vi "test-Mecanum-Kinematics-Test1.vi"() -> (3 "All tests passed":bool)   [LabVIEW 2019]
uses:
  <vilib>/Rock Robotics/WPI/ThirdParty/JAS_Junk/TrajLib/Trajectory_Library.lvlib
panel:
  out "Test 13":bool
  out "Test 12":bool
  out "Test 11":bool
  out "Test 10":bool
  out "Test 9":bool
  out "Test 8":bool
  out "Test 7":bool
  out "Test 6":bool
  out "Test 5":bool
  out "Test 4":bool
  out "Test 3":bool
  out "Test 2":bool
  out "Test 1":bool
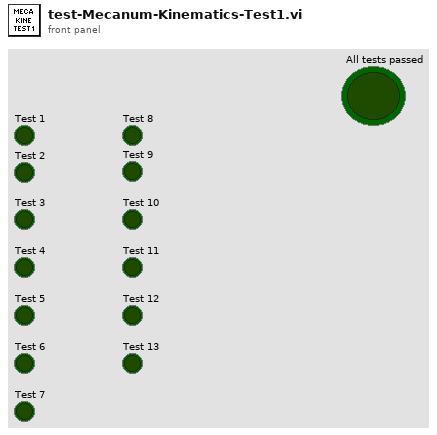
[diagram p1: front panel]
types:
  T1 = typedef "Trajectory_Library.lvlib/TRANSLATION2D.ctl" = cluster{"X":dbl, "Y":dbl}
  T2 = typedef "Trajectory_Library.lvlib/MECA_WHEEL_SPEEDS.ctl" = cluster{"FrontLeftSpeed":dbl, "FrontRightSpeed":dbl, "RearLeftSpeed":dbl, "RearRightSpeed":dbl}
  T3 = typedef "Trajectory_Library.lvlib/CHASSIS_SPEEDS.ctl" = cluster{"vX":dbl, "vY":dbl, "vOmega":dbl}
  T4 = typedef "Trajectory_Library.lvlib/MECA_DRIVE_KINEMATICS.ctl" = cluster{"FrontLeft":T1, "FrontRight":T1, "RearLeft":T1, "RearRight":T1, "InverseKinematics":T5, "ForwardKinematics":T5, "PrevCoR":T1}
  T5 = typedef "NI_Matrix.lvlib/RealMatrix.ctl" = dbl[][]
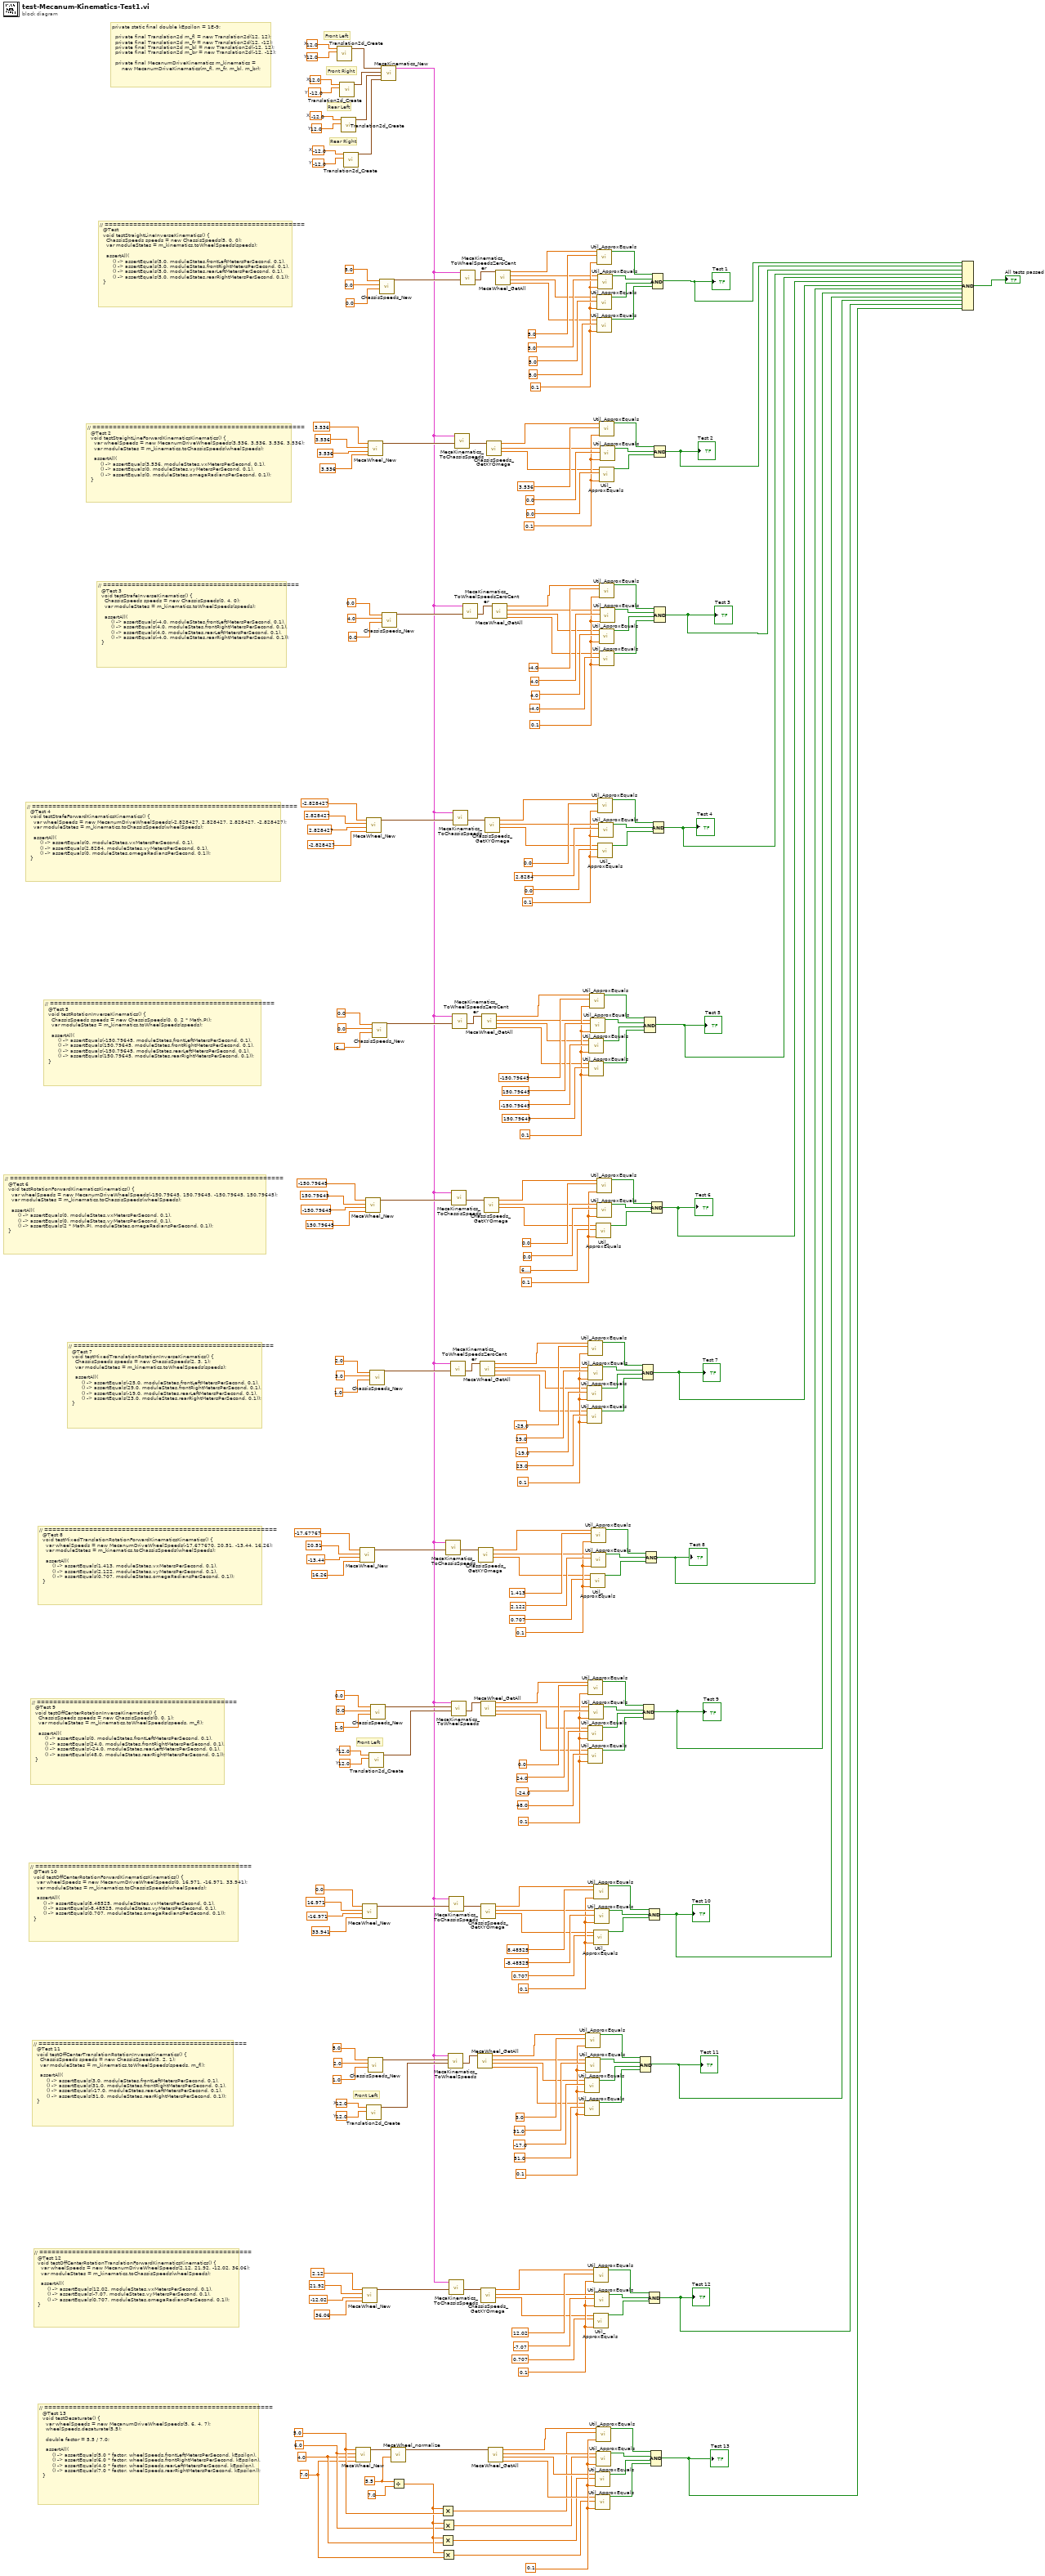
[diagram p0: block diagram]
diagram:
  w11 = 0.1 ("Tolerance")
  w22 = 5.5 ("MaxAttainableSpeed")
  w20 = 5.0 ("FrontLeftSpeed")
  w18 = 6.0 ("FrontRightSpeed")
  w17 = 4.0 ("RearLeftSpeed")
  w16 = 7.0 ("RearRightSpeed")
  w30 = 0.1 ("Tolerance")
  w46 = 12.0  # X
  w44 = 12.0  # Y
  w53 = 0.1 ("Tolerance")
  w67 = 0.1 ("Tolerance")
  w84 = 12.0  # X
  w82 = 12.0  # Y
  w91 = 0.1 ("Tolerance")
  w111 = 0.1 ("Tolerance")
  w131 = 0.1 ("Tolerance")
  w145 = 0.1 ("Tolerance")
  w165 = 0.1 ("Tolerance")
  w178 = 0.1 ("Tolerance")
  w204 = 0.1 ("Tolerance")
  w205 = 0.1 ("Tolerance")
  w206 = 0.1 ("Tolerance")
  w251 = -12.0  # X
  w250 = -12.0  # Y
  w249 = -12.0  # X
  w248 = 12.0  # Y
  w247 = 12.0  # X
  w246 = -12.0  # Y
  w245 = 12.0  # X
  w244 = 12.0  # Y
  # "// ========================================================\n  @Test 13\n  void testDesaturate() {\n    var wheelSpeeds = new MecanumDriveWheelSpeeds(5, 6, 4, 7);\n    wheelSpeeds.desaturate(5.5);\n\n    double factor = 5.5 / 7.0;\n\n    assertAll(\n        () -> assertEquals(5.0 * factor, wheelSpeeds.frontLeftMetersPerSecond, kEpsilon),\n        () -> assertEquals(6.0 * factor, wheelSpeeds.frontRightMetersPerSecond, kEpsilon),\n        () -> assertEquals(4.0 * factor, wheelSpeeds.rearLeftMetersPerSecond, kEpsilon),\n        () -> assertEquals(7.0 * factor, wheelSpeeds.rearRightMetersPerSecond, kEpsilon));\n  }"
  # "// ====================================================\n  @Test 12\n  void testOffCenterRotationTranslationForwardKinematicsKinematics() {\n    var wheelSpeeds = new MecanumDriveWheelSpeeds(2.12, 21.92, -12.02, 36.06);\n    var moduleStates = m_kinematics.toChassisSpeeds(wheelSpeeds);\n\n    assertAll(\n        () -> assertEquals(12.02, moduleStates.vxMetersPerSecond, 0.1),\n        () -> assertEquals(-7.07, moduleStates.vyMetersPerSecond, 0.1),\n        () -> assertEquals(0.707, moduleStates.omegaRadiansPerSecond, 0.1));\n  }"
  # "// ===================================================\n  @Test 11\n  void testOffCenterTranslationRotationInverseKinematics() {\n    ChassisSpeeds speeds = new ChassisSpeeds(5, 2, 1);\n    var moduleStates = m_kinematics.toWheelSpeeds(speeds, m_fl);\n\n    assertAll(\n        () -> assertEquals(3.0, moduleStates.frontLeftMetersPerSecond, 0.1),\n        () -> assertEquals(31.0, moduleStates.frontRightMetersPerSecond, 0.1),\n        () -> assertEquals(-17.0, moduleStates.rearLeftMetersPerSecond, 0.1),\n        () -> assertEquals(51.0, moduleStates.rearRightMetersPerSecond, 0.1));\n  }"
  # "Front Left"
  # "// =====================================================\n  @Test 10\n  void testOffCenterRotationForwardKinematicsKinematics() {\n    var wheelSpeeds = new MecanumDriveWheelSpeeds(0, 16.971, -16.971, 33.941);\n    var moduleStates = m_kinematics.toChassisSpeeds(wheelSpeeds);\n\n    assertAll(\n        () -> assertEquals(8.48525, moduleStates.vxMetersPerSecond, 0.1),\n        () -> assertEquals(-8.48525, moduleStates.vyMetersPerSecond, 0.1),\n        () -> assertEquals(0.707, moduleStates.omegaRadiansPerSecond, 0.1));\n  }"
  # "Front Left"
  # "// =================================================\n  @Test 9\n  void testOffCenterRotationInverseKinematics() {\n    ChassisSpeeds speeds = new ChassisSpeeds(0, 0, 1);\n    var moduleStates = m_kinematics.toWheelSpeeds(speeds, m_fl);\n\n    assertAll(\n        () -> assertEquals(0, moduleStates.frontLeftMetersPerSecond, 0.1),\n        () -> assertEquals(24.0, moduleStates.frontRightMetersPerSecond, 0.1),\n        () -> assertEquals(-24.0, moduleStates.rearLeftMetersPerSecond, 0.1),\n        () -> assertEquals(48.0, moduleStates.rearRightMetersPerSecond, 0.1));\n  }"
  # "// =========================================================\n  @Test 8\n  void testMixedTranslationRotationForwardKinematicsKinematics() {\n    var wheelSpeeds = new MecanumDriveWheelSpeeds(-17.677670, 20.51, -13.44, 16.26);\n    var moduleStates = m_kinematics.toChassisSpeeds(wheelSpeeds);\n\n    assertAll(\n        () -> assertEquals(1.413, moduleStates.vxMetersPerSecond, 0.1),\n        () -> assertEquals(2.122, moduleStates.vyMetersPerSecond, 0.1),\n        () -> assertEquals(0.707, moduleStates.omegaRadiansPerSecond, 0.1));\n  }"
  # "// =================================================\n  @Test 7\n  void testMixedTranslationRotationInverseKinematics() {\n    ChassisSpeeds speeds = new ChassisSpeeds(2, 3, 1);\n    var moduleStates = m_kinematics.toWheelSpeeds(speeds);\n\n    assertAll(\n        () -> assertEquals(-25.0, moduleStates.frontLeftMetersPerSecond, 0.1),\n        () -> assertEquals(29.0, moduleStates.frontRightMetersPerSecond, 0.1),\n        () -> assertEquals(-19.0, moduleStates.rearLeftMetersPerSecond, 0.1),\n        () -> assertEquals(23.0, moduleStates.rearRightMetersPerSecond, 0.1));\n  }"
  # "// ===================================================================\n  @Test 6\n  void testRotationForwardKinematicsKinematics() {\n    var wheelSpeeds = new MecanumDriveWheelSpeeds(-150.79645, 150.79645, -150.79645, 150.79645);\n    var moduleStates = m_kinematics.toChassisSpeeds(wheelSpeeds);\n\n    assertAll(\n        () -> assertEquals(0, moduleStates.vxMetersPerSecond, 0.1),\n        () -> assertEquals(0, moduleStates.vyMetersPerSecond, 0.1),\n        () -> assertEquals(2 * Math.PI, moduleStates.omegaRadiansPerSecond, 0.1));\n  }"
  # "// =======================================================\n  @Test 5\n  void testRotationInverseKinematics() {\n    ChassisSpeeds speeds = new ChassisSpeeds(0, 0, 2 * Math.PI);\n    var moduleStates = m_kinematics.toWheelSpeeds(speeds);\n\n    assertAll(\n        () -> assertEquals(-150.79645, moduleStates.frontLeftMetersPerSecond, 0.1),\n        () -> assertEquals(150.79645, moduleStates.frontRightMetersPerSecond, 0.1),\n        () -> assertEquals(-150.79645, moduleStates.rearLeftMetersPerSecond, 0.1),\n        () -> assertEquals(150.79645, moduleStates.rearRightMetersPerSecond, 0.1));\n  }"
  # "// =================================================================\n  @Test 4\n  void testStrafeForwardKinematicsKinematics() {\n    var wheelSpeeds = new MecanumDriveWheelSpeeds(-2.828427, 2.828427, 2.828427, -2.828427);\n    var moduleStates = m_kinematics.toChassisSpeeds(wheelSpeeds);\n\n    assertAll(\n        () -> assertEquals(0, moduleStates.vxMetersPerSecond, 0.1),\n        () -> assertEquals(2.8284, moduleStates.vyMetersPerSecond, 0.1),\n        () -> assertEquals(0, moduleStates.omegaRadiansPerSecond, 0.1));\n  }"
  # "// ================================================\n  @Test 3\n  void testStrafeInverseKinematics() {\n    ChassisSpeeds speeds = new ChassisSpeeds(0, 4, 0);\n    var moduleStates = m_kinematics.toWheelSpeeds(speeds);\n\n    assertAll(\n        () -> assertEquals(-4.0, moduleStates.frontLeftMetersPerSecond, 0.1),\n        () -> assertEquals(4.0, moduleStates.frontRightMetersPerSecond, 0.1),\n        () -> assertEquals(4.0, moduleStates.rearLeftMetersPerSecond, 0.1),\n        () -> assertEquals(-4.0, moduleStates.rearRightMetersPerSecond, 0.1));\n  }"
  # "// ====================================================\n  @Test 2\n  void testStraightLineForwardKinematicsKinematics() {\n    var wheelSpeeds = new MecanumDriveWheelSpeeds(3.536, 3.536, 3.536, 3.536);\n    var moduleStates = m_kinematics.toChassisSpeeds(wheelSpeeds);\n\n    assertAll(\n        () -> assertEquals(3.536, moduleStates.vxMetersPerSecond, 0.1),\n        () -> assertEquals(0, moduleStates.vyMetersPerSecond, 0.1),\n        () -> assertEquals(0, moduleStates.omegaRadiansPerSecond, 0.1));\n  }"
  # "Rear Right"
  # "Rear Left"
  # "Front Right"
  # "Front Left"
  # "private static final double kEpsilon = 1E-9;\n\n  private final Translation2d m_fl = new Translation2d(12, 12);\n  private final Translation2d m_fr = new Translation2d(12, -12);\n  private final Translation2d m_bl = new Translation2d(-12, 12);\n  private final Translation2d m_br = new Translation2d(-12, -12);\n\n  private final MecanumDriveKinematics m_kinematics =\n      new MecanumDriveKinematics(m_fl, m_fr, m_bl, m_br);"
  # "// =================================================\n  @Test\n  void testStraightLineInverseKinematics() {\n    ChassisSpeeds speeds = new ChassisSpeeds(5, 0, 0);\n    var moduleStates = m_kinematics.toWheelSpeeds(speeds);\n\n    assertAll(\n        () -> assertEquals(5.0, moduleStates.frontLeftMetersPerSecond, 0.1),\n        () -> assertEquals(5.0, moduleStates.frontRightMetersPerSecond, 0.1),\n        () -> assertEquals(5.0, moduleStates.rearLeftMetersPerSecond, 0.1),\n        () -> assertEquals(5.0, moduleStates.rearRightMetersPerSecond, 0.1));\n  }"
  n1 = call <vilib>:"Translation2d_Create.vi"("Y"=w244, "X"=w245) -> ("TRANSLATION"=w252:T1)  [unwired: 9 in]
  n2 = call <vilib>:"Translation2d_Create.vi"("Y"=w246, "X"=w247) -> ("TRANSLATION"=w253:T1)  [unwired: 9 in]
  n3 = call <vilib>:"Translation2d_Create.vi"("Y"=w248, "X"=w249) -> ("TRANSLATION"=w254:T1)  [unwired: 9 in]
  n4 = call <vilib>:"Translation2d_Create.vi"("Y"=w250, "X"=w251) -> ("TRANSLATION"=w255:T1)  [unwired: 9 in]
  n5 = call <vilib>:"MecaWheel_New.vi"("RearRightSpeed"=w16, "RearLeftSpeed"=w17, "FrontRightSpeed"=w18, "FrontLeftSpeed"=w20) -> ("MECA_WHEEL_SPEEDS"=w23:T2)  [unwired: 7 in]
  n6 = call <vilib>:"MecaWheel_New.vi"("RearRightSpeed"=16.26, "RearLeftSpeed"=-13.44, "FrontRightSpeed"=20.51, "FrontLeftSpeed"=-17.67767) -> ("MECA_WHEEL_SPEEDS"=w115:T2)  [unwired: 7 in]
  n7 = call <vilib>:"MecaWheel_New.vi"("RearRightSpeed"=33.941, "RearLeftSpeed"=-16.971, "FrontRightSpeed"=16.971, "FrontLeftSpeed"=0.0) -> ("MECA_WHEEL_SPEEDS"=w71:T2)  [unwired: 7 in]
  n8 = call <vilib>:"MecaWheel_New.vi"("RearRightSpeed"=36.06, "RearLeftSpeed"=-12.02, "FrontRightSpeed"=21.92, "FrontLeftSpeed"=2.12) -> ("MECA_WHEEL_SPEEDS"=w34:T2)  [unwired: 7 in]
  n9 = call <vilib>:"MecaWheel_New.vi"("RearRightSpeed"=150.79645, "RearLeftSpeed"=-150.79645, "FrontRightSpeed"=150.79645, "FrontLeftSpeed"=-150.79645) -> ("MECA_WHEEL_SPEEDS"=w149:T2)  [unwired: 7 in]
  n10 = call <vilib>:"Translation2d_Create.vi"("Y"=w44, "X"=w46) -> ("TRANSLATION"=w45:T1)  [unwired: 9 in]
  n11 = call <vilib>:"MecaWheel_New.vi"("RearRightSpeed"=-2.828427, "RearLeftSpeed"=2.828427, "FrontRightSpeed"=2.828427, "FrontLeftSpeed"=-2.828427) -> ("MECA_WHEEL_SPEEDS"=w182:T2)  [unwired: 7 in]
  n12 = call <vilib>:"ChassisSpeeds_New.vi"("vAngular"=1.0 ("vX"), "vY"=2.0, "vX"=5.0) -> ("CHASSIS"=w27:T3)  [unwired: 8 in]
  n13 = call <vilib>:"MecaWheel_New.vi"("RearRightSpeed"=3.536, "RearLeftSpeed"=3.536, "FrontRightSpeed"=3.536, "FrontLeftSpeed"=3.536) -> ("MECA_WHEEL_SPEEDS"=w223:T2)  [unwired: 7 in]
  n14 = call <vilib>:"Translation2d_Create.vi"("Y"=w82, "X"=w84) -> ("TRANSLATION"=w83:T1)  [unwired: 9 in]
  n15 = call <vilib>:"ChassisSpeeds_New.vi"("vAngular"=1.0 ("vX"), "vY"=3.0, "vX"=2.0) -> ("CHASSIS"=w140:T3)  [unwired: 8 in]
  n16 = call <vilib>:"ChassisSpeeds_New.vi"("vAngular"=1.0 ("vX"), "vY"=0.0, "vX"=0.0) -> ("CHASSIS"=w100:T3)  [unwired: 8 in]
  n17 = call <vilib>:"ChassisSpeeds_New.vi"("vAngular"=6.283185307179586, "vY"=0.0, "vX"=0.0) -> ("CHASSIS"=w174:T3)  [unwired: 8 in]
  n18 = call <vilib>:"ChassisSpeeds_New.vi"("vAngular"=0.0, "vY"=0.0, "vX"=5.0) -> ("CHASSIS"=w243:T3)  [unwired: 8 in]
  n19 = call <vilib>:"MecaKinematics_New.vi"("RearRight"=w255, "RearLeft"=w254, "FrontRight"=w253, "FrontLeft"=w252) -> ("MECA_DRIVE_KINEMATICS"=w26:T4)  [unwired: 7 in]
  n20 = call <vilib>:"ChassisSpeeds_New.vi"("vAngular"=0.0, "vY"=4.0, "vX"=0.0) -> ("CHASSIS"=w215:T3)  [unwired: 8 in]
  n21 = call <vilib>:"MecaWheel_normalize.vi"("MaxAttainableSpeed"=w22, "in MECA_WHEEL_SPEEDS"=w23) -> ("out MECA_WHEEL_SPEEDS"=w6:T2)  [unwired: 9 in]
  n22 = Divide(x=w22, y=7.0) -> (x/y=w19:dbl)
  n23 = Multiply(x=w19, y=w20) -> (x*y=w5:dbl)
  n24 = Multiply(x=w19, y=w17) -> (x*y=w3:dbl)
  n25 = Multiply(x=w19, y=w18) -> (x*y=w4:dbl)
  n26 = Multiply(x=w19, y=w16) -> (x*y=w2:dbl)
  n27 = call <vilib>:"MecaKinematics_ToChassisSpeeds.vi"("MECA_WHEEL_SPEEDS"=w115, "in MECA_DRIVE_KINEMATICS"=w26) -> ("ChassisSpeeds"=w114:T3)  [unwired: 9 in]
  n28 = call <vilib>:"MecaKinematics_ToWheelSpeeds.vi"("CenterOfRotation"=w45, "ChassisSpeeds"=w27, "in MECA_DRIVE_KINEMATICS"=w26) -> ("MECA_WHEEL_SPEEDS"=w52:T2)  [unwired: 7 in, 1 out]
  n29 = call <vilib>:"MecaKinematics_ToChassisSpeeds.vi"("MECA_WHEEL_SPEEDS"=w71, "in MECA_DRIVE_KINEMATICS"=w26) -> ("ChassisSpeeds"=w70:T3)  [unwired: 9 in]
  n30 = call <vilib>:"MecaKinematics_ToChassisSpeeds.vi"("MECA_WHEEL_SPEEDS"=w34, "in MECA_DRIVE_KINEMATICS"=w26) -> ("ChassisSpeeds"=w33:T3)  [unwired: 9 in]
  n31 = call <vilib>:"MecaKinematics_ToWheelSpeedsZeroCenter.vi"("ChassisSpeeds"=w140, "in MECA_DRIVE_KINEMATICS"=w26) -> ("MECA_WHEEL_SPEEDS"=w130:T2)  [unwired: 8 in, 1 out]
  n32 = call <vilib>:"MecaKinematics_ToWheelSpeeds.vi"("CenterOfRotation"=w83, "ChassisSpeeds"=w100, "in MECA_DRIVE_KINEMATICS"=w26) -> ("MECA_WHEEL_SPEEDS"=w90:T2)  [unwired: 7 in, 1 out]
  n33 = call <vilib>:"MecaKinematics_ToChassisSpeeds.vi"("MECA_WHEEL_SPEEDS"=w149, "in MECA_DRIVE_KINEMATICS"=w26) -> ("ChassisSpeeds"=w148:T3)  [unwired: 9 in]
  n34 = call <vilib>:"MecaKinematics_ToWheelSpeedsZeroCenter.vi"("ChassisSpeeds"=w174, "in MECA_DRIVE_KINEMATICS"=w26) -> ("MECA_WHEEL_SPEEDS"=w164:T2)  [unwired: 8 in, 1 out]
  n35 = call <vilib>:"MecaKinematics_ToChassisSpeeds.vi"("MECA_WHEEL_SPEEDS"=w182, "in MECA_DRIVE_KINEMATICS"=w26) -> ("ChassisSpeeds"=w181:T3)  [unwired: 9 in]
  n36 = call <vilib>:"MecaKinematics_ToChassisSpeeds.vi"("MECA_WHEEL_SPEEDS"=w223, "in MECA_DRIVE_KINEMATICS"=w26) -> ("ChassisSpeeds"=w222:T3)  [unwired: 9 in]
  n37 = call <vilib>:"MecaKinematics_ToWheelSpeedsZeroCenter.vi"("ChassisSpeeds"=w243, "in MECA_DRIVE_KINEMATICS"=w26) -> ("MECA_WHEEL_SPEEDS"=w203:T2)  [unwired: 8 in, 1 out]
  n38 = call <vilib>:"MecaKinematics_ToWheelSpeedsZeroCenter.vi"("ChassisSpeeds"=w215, "in MECA_DRIVE_KINEMATICS"=w26) -> ("MECA_WHEEL_SPEEDS"=w198:T2)  [unwired: 8 in, 1 out]
  n39 = call <vilib>:"MecaWheel_GetAll.vi"("MECA_WHEEL_SPEEDS"=w52) -> ("RearRightSpeed"=w48:dbl, "RearLeftSpeed"=w49:dbl, "FrontRightSpeed"=w50:dbl, "FrontLeftSpeed"=w51:dbl)  [unwired: 7 in]
  n40 = call <vilib>:"ChassisSpeeds_GetXYOmega.vi"("CHASSIS"=w114) -> ("vAngular"=w110:dbl, "vY"=w112:dbl, "vX"=w113:dbl)  [unwired: 8 in]
  n41 = call <vilib>:"MecaWheel_GetAll.vi"("MECA_WHEEL_SPEEDS"=w130) -> ("RearRightSpeed"=w126:dbl, "RearLeftSpeed"=w127:dbl, "FrontRightSpeed"=w128:dbl, "FrontLeftSpeed"=w129:dbl)  [unwired: 7 in]
  n42 = call <vilib>:"MecaWheel_GetAll.vi"("MECA_WHEEL_SPEEDS"=w90) -> ("RearRightSpeed"=w86:dbl, "RearLeftSpeed"=w87:dbl, "FrontRightSpeed"=w88:dbl, "FrontLeftSpeed"=w89:dbl)  [unwired: 7 in]
  n43 = call <vilib>:"ChassisSpeeds_GetXYOmega.vi"("CHASSIS"=w70) -> ("vAngular"=w66:dbl, "vY"=w68:dbl, "vX"=w69:dbl)  [unwired: 8 in]
  n44 = call <vilib>:"ChassisSpeeds_GetXYOmega.vi"("CHASSIS"=w33) -> ("vAngular"=w29:dbl, "vY"=w31:dbl, "vX"=w32:dbl)  [unwired: 8 in]
  n45 = call <vilib>:"MecaWheel_GetAll.vi"("MECA_WHEEL_SPEEDS"=w164) -> ("RearRightSpeed"=w160:dbl, "RearLeftSpeed"=w161:dbl, "FrontRightSpeed"=w162:dbl, "FrontLeftSpeed"=w163:dbl)  [unwired: 7 in]
  n46 = call <vilib>:"ChassisSpeeds_GetXYOmega.vi"("CHASSIS"=w148) -> ("vAngular"=w144:dbl, "vY"=w146:dbl, "vX"=w147:dbl)  [unwired: 8 in]
  n47 = call <vilib>:"ChassisSpeeds_GetXYOmega.vi"("CHASSIS"=w181) -> ("vAngular"=w177:dbl, "vY"=w179:dbl, "vX"=w180:dbl)  [unwired: 8 in]
  n48 = call <vilib>:"ChassisSpeeds_GetXYOmega.vi"("CHASSIS"=w222) -> ("vAngular"=w193:dbl, "vY"=w220:dbl, "vX"=w221:dbl)  [unwired: 8 in]
  n49 = call <vilib>:"MecaWheel_GetAll.vi"("MECA_WHEEL_SPEEDS"=w6) -> ("RearRightSpeed"=w7:dbl, "RearLeftSpeed"=w8:dbl, "FrontRightSpeed"=w9:dbl, "FrontLeftSpeed"=w10:dbl)  [unwired: 7 in]
  n50 = call <vilib>:"MecaWheel_GetAll.vi"("MECA_WHEEL_SPEEDS"=w198) -> ("RearRightSpeed"=w194:dbl, "RearLeftSpeed"=w195:dbl, "FrontRightSpeed"=w196:dbl, "FrontLeftSpeed"=w197:dbl)  [unwired: 7 in]
  n51 = call <vilib>:"MecaWheel_GetAll.vi"("MECA_WHEEL_SPEEDS"=w203) -> ("RearRightSpeed"=w199:dbl, "RearLeftSpeed"=w200:dbl, "FrontRightSpeed"=w201:dbl, "FrontLeftSpeed"=w202:dbl)  [unwired: 7 in]
  n52 = call <vilib>:"Util_ApproxEquals.vi"("Tolerance"=w53, "Value 2"=-17.0, "Value 1"=w49) -> ("ApproxEquals"=w55:bool)  [unwired: 8 in]
  n53 = call <vilib>:"Util_ApproxEquals.vi"("Tolerance"=w53, "Value 2"=51.0, "Value 1"=w48) -> ("ApproxEquals"=w54:bool)  [unwired: 8 in]
  n54 = call <vilib>:"Util_ApproxEquals.vi"("Tolerance"=w53, "Value 2"=3.0, "Value 1"=w51) -> ("ApproxEquals"=w57:bool)  [unwired: 8 in]
  n55 = call <vilib>:"Util_ApproxEquals.vi"("Tolerance"=w53, "Value 2"=31.0, "Value 1"=w50) -> ("ApproxEquals"=w56:bool)  [unwired: 8 in]
  n56 = call <vilib>:"Util_ApproxEquals.vi"("Tolerance"=w131, "Value 2"=-19.0, "Value 1"=w127) -> ("ApproxEquals"=w133:bool)  [unwired: 8 in]
  n57 = call <vilib>:"Util_ApproxEquals.vi"("Tolerance"=w131, "Value 2"=23.0, "Value 1"=w126) -> ("ApproxEquals"=w132:bool)  [unwired: 8 in]
  n58 = call <vilib>:"Util_ApproxEquals.vi"("Tolerance"=w131, "Value 2"=-25.0, "Value 1"=w129) -> ("ApproxEquals"=w135:bool)  [unwired: 8 in]
  n59 = call <vilib>:"Util_ApproxEquals.vi"("Tolerance"=w91, "Value 2"=-24.0, "Value 1"=w87) -> ("ApproxEquals"=w93:bool)  [unwired: 8 in]
  n60 = call <vilib>:"Util_ApproxEquals.vi"("Tolerance"=w91, "Value 2"=48.0, "Value 1"=w86) -> ("ApproxEquals"=w92:bool)  [unwired: 8 in]
  n61 = call <vilib>:"Util_ApproxEquals.vi"("Tolerance"=w131, "Value 2"=29.0, "Value 1"=w128) -> ("ApproxEquals"=w134:bool)  [unwired: 8 in]
  n62 = call <vilib>:"Util_ApproxEquals.vi"("Tolerance"=w91, "Value 2"=0.0, "Value 1"=w89) -> ("ApproxEquals"=w95:bool)  [unwired: 8 in]
  n63 = call <vilib>:"Util_ApproxEquals.vi"("Tolerance"=w91, "Value 2"=24.0, "Value 1"=w88) -> ("ApproxEquals"=w94:bool)  [unwired: 8 in]
  n64 = call <vilib>:"Util_ApproxEquals.vi"("Tolerance"=w165, "Value 2"=-150.79645, "Value 1"=w161) -> ("ApproxEquals"=w167:bool)  [unwired: 8 in]
  n65 = call <vilib>:"Util_ApproxEquals.vi"("Tolerance"=w165, "Value 2"=150.79645, "Value 1"=w160) -> ("ApproxEquals"=w166:bool)  [unwired: 8 in]
  n66 = call <vilib>:"Util_ApproxEquals.vi"("Tolerance"=w165, "Value 2"=-150.79645, "Value 1"=w163) -> ("ApproxEquals"=w169:bool)  [unwired: 8 in]
  n67 = call <vilib>:"Util_ApproxEquals.vi"("Tolerance"=w165, "Value 2"=150.79645, "Value 1"=w162) -> ("ApproxEquals"=w168:bool)  [unwired: 8 in]
  n68 = call <vilib>:"Util_ApproxEquals.vi"("Tolerance"=w111, "Value 2"=0.707, "Value 1"=w110) -> ("ApproxEquals"=w120:bool)  [unwired: 8 in]
  n69 = call <vilib>:"Util_ApproxEquals.vi"("Tolerance"=w111, "Value 2"=1.413, "Value 1"=w113) -> ("ApproxEquals"=w122:bool)  [unwired: 8 in]
  n70 = call <vilib>:"Util_ApproxEquals.vi"("Tolerance"=w111, "Value 2"=2.122, "Value 1"=w112) -> ("ApproxEquals"=w121:bool)  [unwired: 8 in]
  n71 = call <vilib>:"Util_ApproxEquals.vi"("Tolerance"=w67, "Value 2"=0.707, "Value 1"=w66) -> ("ApproxEquals"=w76:bool)  [unwired: 8 in]
  n72 = call <vilib>:"Util_ApproxEquals.vi"("Tolerance"=w30, "Value 2"=0.707, "Value 1"=w29) -> ("ApproxEquals"=w39:bool)  [unwired: 8 in]
  n73 = call <vilib>:"Util_ApproxEquals.vi"("Tolerance"=w67, "Value 2"=8.48525, "Value 1"=w69) -> ("ApproxEquals"=w78:bool)  [unwired: 8 in]
  n74 = call <vilib>:"Util_ApproxEquals.vi"("Tolerance"=w30, "Value 2"=12.02, "Value 1"=w32) -> ("ApproxEquals"=w41:bool)  [unwired: 8 in]
  n75 = call <vilib>:"Util_ApproxEquals.vi"("Tolerance"=w67, "Value 2"=-8.48525, "Value 1"=w68) -> ("ApproxEquals"=w77:bool)  [unwired: 8 in]
  n76 = call <vilib>:"Util_ApproxEquals.vi"("Tolerance"=w30, "Value 2"=-7.07, "Value 1"=w31) -> ("ApproxEquals"=w40:bool)  [unwired: 8 in]
  n77 = call <vilib>:"Util_ApproxEquals.vi"("Tolerance"=w11, "Value 2"=w3, "Value 1"=w8) -> ("ApproxEquals"=w13:bool)  [unwired: 8 in]
  n78 = call <vilib>:"Util_ApproxEquals.vi"("Tolerance"=w11, "Value 2"=w2, "Value 1"=w7) -> ("ApproxEquals"=w12:bool)  [unwired: 8 in]
  n79 = call <vilib>:"Util_ApproxEquals.vi"("Tolerance"=w11, "Value 2"=w5, "Value 1"=w10) -> ("ApproxEquals"=w15:bool)  [unwired: 8 in]
  n80 = call <vilib>:"Util_ApproxEquals.vi"("Tolerance"=w145, "Value 2"=6.283185307179586, "Value 1"=w144) -> ("ApproxEquals"=w154:bool)  [unwired: 8 in]
  n81 = call <vilib>:"Util_ApproxEquals.vi"("Tolerance"=w11, "Value 2"=w4, "Value 1"=w9) -> ("ApproxEquals"=w14:bool)  [unwired: 8 in]
  n82 = call <vilib>:"Util_ApproxEquals.vi"("Tolerance"=w206, "Value 2"=5.0, "Value 1"=w200) -> ("ApproxEquals"=w236:bool)  [unwired: 8 in]
  n83 = call <vilib>:"Util_ApproxEquals.vi"("Tolerance"=w206, "Value 2"=5.0, "Value 1"=w199) -> ("ApproxEquals"=w235:bool)  [unwired: 8 in]
  n84 = call <vilib>:"Util_ApproxEquals.vi"("Tolerance"=w145, "Value 2"=0.0, "Value 1"=w147) -> ("ApproxEquals"=w156:bool)  [unwired: 8 in]
  n85 = call <vilib>:"Util_ApproxEquals.vi"("Tolerance"=w206, "Value 2"=5.0, "Value 1"=w202) -> ("ApproxEquals"=w238:bool)  [unwired: 8 in]
  n86 = call <vilib>:"Util_ApproxEquals.vi"("Tolerance"=w145, "Value 2"=0.0, "Value 1"=w146) -> ("ApproxEquals"=w155:bool)  [unwired: 8 in]
  n87 = call <vilib>:"Util_ApproxEquals.vi"("Tolerance"=w206, "Value 2"=5.0, "Value 1"=w201) -> ("ApproxEquals"=w237:bool)  [unwired: 8 in]
  n88 = call <vilib>:"Util_ApproxEquals.vi"("Tolerance"=w178, "Value 2"=0.0, "Value 1"=w177) -> ("ApproxEquals"=w187:bool)  [unwired: 8 in]
  n89 = call <vilib>:"Util_ApproxEquals.vi"("Tolerance"=w178, "Value 2"=0.0, "Value 1"=w180) -> ("ApproxEquals"=w189:bool)  [unwired: 8 in]
  n90 = call <vilib>:"Util_ApproxEquals.vi"("Tolerance"=w178, "Value 2"=2.8284, "Value 1"=w179) -> ("ApproxEquals"=w188:bool)  [unwired: 8 in]
  n91 = call <vilib>:"Util_ApproxEquals.vi"("Tolerance"=w205, "Value 2"=0.0, "Value 1"=w193) -> ("ApproxEquals"=w228:bool)  [unwired: 8 in]
  n92 = call <vilib>:"Util_ApproxEquals.vi"("Tolerance"=w204, "Value 2"=4.0, "Value 1"=w195) -> ("ApproxEquals"=w208:bool)  [unwired: 8 in]
  n93 = call <vilib>:"Util_ApproxEquals.vi"("Tolerance"=w204, "Value 2"=-4.0, "Value 1"=w194) -> ("ApproxEquals"=w207:bool)  [unwired: 8 in]
  n94 = call <vilib>:"Util_ApproxEquals.vi"("Tolerance"=w205, "Value 2"=3.536, "Value 1"=w221) -> ("ApproxEquals"=w230:bool)  [unwired: 8 in]
  n95 = call <vilib>:"Util_ApproxEquals.vi"("Tolerance"=w204, "Value 2"=-4.0, "Value 1"=w197) -> ("ApproxEquals"=w210:bool)  [unwired: 8 in]
  n96 = call <vilib>:"Util_ApproxEquals.vi"("Tolerance"=w205, "Value 2"=0.0, "Value 1"=w220) -> ("ApproxEquals"=w229:bool)  [unwired: 8 in]
  n97 = call <vilib>:"Util_ApproxEquals.vi"("Tolerance"=w204, "Value 2"=4.0, "Value 1"=w196) -> ("ApproxEquals"=w209:bool)  [unwired: 8 in]
  n98 = Compound Arithmetic op=AND(w57, w56, w55, w54) -> (w25:bool)
  "Test 11" <- w25
  n99 = Compound Arithmetic op=AND(w135, w134, w133, w132) -> (w104:bool)
  "Test 7" <- w104
  n100 = Compound Arithmetic op=AND(w95, w94, w93, w92) -> (w81:bool)
  "Test 9" <- w81
  n101 = Compound Arithmetic op=AND(w169, w168, w167, w166) -> (w106:bool)
  "Test 5" <- w106
  n102 = Compound Arithmetic op=AND(w122, w121, w120) -> (w103:bool)
  "Test 8" <- w103
  n103 = Compound Arithmetic op=AND(w78, w77, w76) -> (w64:bool)
  "Test 10" <- w64
  n104 = Compound Arithmetic op=AND(w41, w40, w39) -> (w24:bool)
  "Test 12" <- w24
  n105 = Compound Arithmetic op=AND(w15, w14, w13, w12) -> (w1:bool)
  "Test 13" <- w1
  n106 = Compound Arithmetic op=AND(w156, w155, w154) -> (w105:bool)
  "Test 6" <- w105
  n107 = Compound Arithmetic op=AND(w238, w237, w236, w235) -> (w234:bool)
  "Test 1" <- w234
  n108 = Compound Arithmetic op=AND(w189, w188, w187) -> (w107:bool)
  "Test 4" <- w107
  n109 = Compound Arithmetic op=AND(w230, w229, w228) -> (w219:bool)
  "Test 2" <- w219
  n110 = Compound Arithmetic op=AND(w210, w209, w208, w207) -> (w108:bool)
  "Test 3" <- w108
  n111 = Compound Arithmetic op=AND(w234, w219, w108, w107, w106, w105, w104, w103, w81, w64, w25, w24, w1) -> (→"All tests passed":bool)
